vi "Tip Voltage.vi"(1 "Output Voltage":dbl format="%_5p") -> (0 "error out":errorcluster)   [LabVIEW 2011]
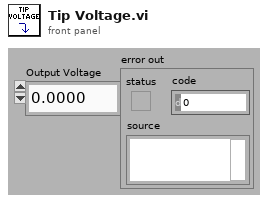
[diagram p1: front panel]
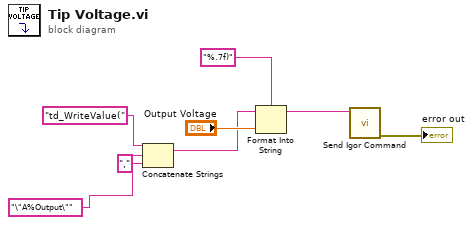
[diagram p0: block diagram]
diagram:
  n1 = Concatenate Strings("td_WriteValue(", "\"A%Output\"", "," ("string")) -> (w5:string)
  n2 = Format Into String "Format Into String"(format string="%.7f)" ("Number resolutio"), initial string=w5, "Output Voltage") -> (resulting string=w3:string)  [unwired: 1 in, 1 out]
  n3 = call "Send Igor Command.vi"("Command"=w3) -> ("error out"=→"error out":errorcluster)  [unwired: 7 in, 2 out]
